vi "2 Steering Chooser.vi"() -> (2 "rudder setpoint":T2=-30.0 format="%05.1f")   [LabVIEW 2011]
doc: "Takes waypoint and boat location information from the global variable and places the approproate rudder position command on the global.\nFor Drive waypoints, this VI simply tries to make the boat's heading the same as the heading between the boat and the waypoint. TODO: this does not account for drift -- it assumes that the boat will go where it is pointed which is not always the case.\n\nTODO: important: As of 11/17 this VI only works for the Drive option.\nTODO: ideally this VI would run on any update of the boat location or waypoint location, and not otherwise."
uses:
  2 Typedefs/heading.ctl
  2 Typedefs/UTM Location.ctl
  2 Typedefs/Velocity.ctl
  2 Classes/Waypoint/Waypoint.lvclass
  2 Globals/2 Global.vi
panel:
  out "Robot UTM Location 2":T1 {"North" format="%#_10f"; "East" format="%#_8f"}
  in  "maximum rudder deflection":T2=-30.0 format="%05.1f"
  out "Robot\nHeading":T2 format="%05.1f"
  out "Angle to waypt":T2 format="%05.1f"
  out "Distance to Waypoint":T3
  out "Robot UTM Location":T1 {"North" format="%#_10f"; "East" format="%#_8f"}
  out "desired delta heading":T2 format="%05.1f"
  # "Steering Chooser simply turns the rudder to aim the boat's bow towards the next waypoint.\n\nTODO: currently only implements Drive waypoints. Also this is extremely stupid.\nImplement avoidance, stay-in-area, and maybe a PID loop."
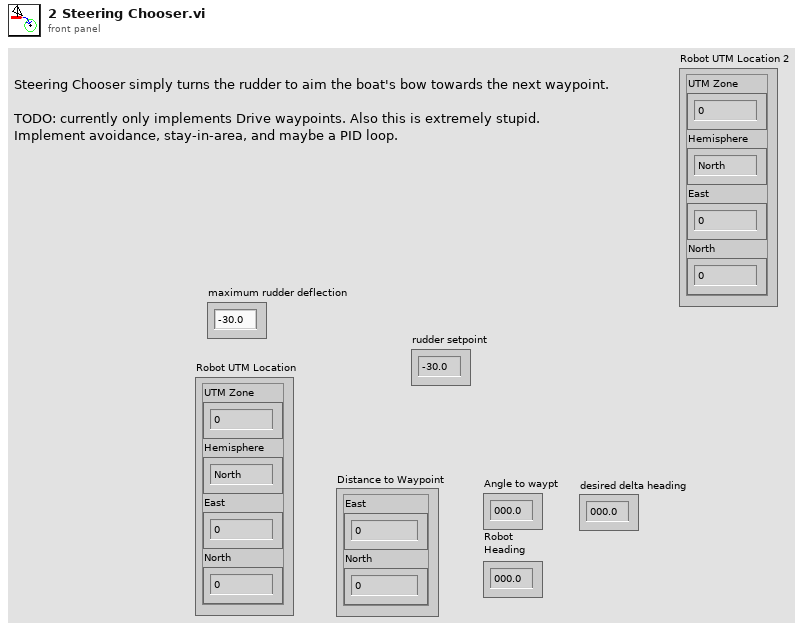
[diagram p1: front panel]
types:
  T1 = typedef "UTM Location.ctl" = cluster{"UTM Zone":dbl, "Hemisphere":enum16{"North", "South"}, "East":dbl, "North":dbl}
  T2 = typedef "heading.ctl" = dbl
  T3 = typedef "Velocity.ctl" = cluster{"East":dbl, "North":dbl}
  T4 = typedef "Current Waypoint.ctl" = i32
  T5 = typedef "Waypoints List.ctl" = refnum<class "Waypoint.lvclass">[]
  T6 = cluster{"UTM Zone":dbl, "Hemisphere":u16, "East":dbl, "North":dbl}
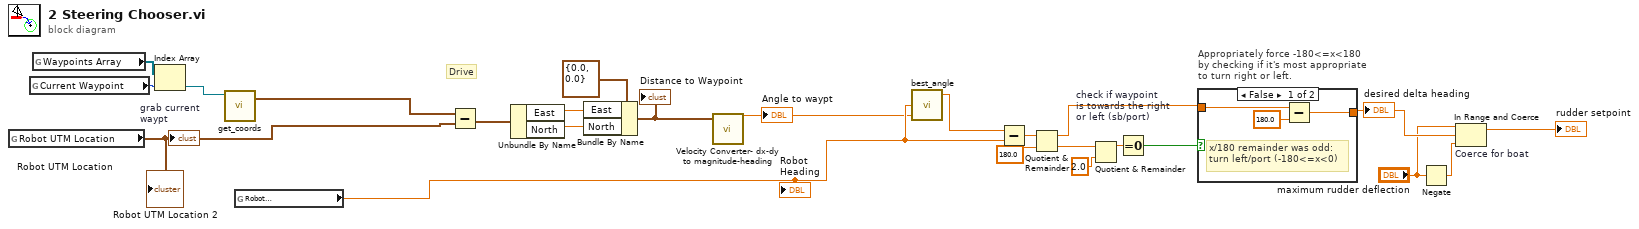
[diagram p0: block diagram]
diagram:
  # "Drive"
  n1 = global read "2 Global.vi" "Robot UTM Location"() -> (w24:T1)
  "Robot UTM Location" <- w24
  "Robot UTM Location 2" <- w24
  n2 = global read "2 Global.vi" "Current Waypoint"() -> (w21:T4)
  n3 = global read "2 Global.vi" "Waypoints Array"() -> (w22:T5)
  n4 = Index Array "grab current\nwaypt"(array=w22, index=w21) -> (element=w20:refnum<class "Waypoint.lvclass">)
  n5 = call-dynamic "get_coords.vi"("Waypoint in"=w20) -> ("Coords"=w19:T1)  [unwired: 7 in, 3 out]
  n6 = global read "2 Global.vi" "Robot\nHeading"() -> (w23:T2)
  "Robot\nHeading" <- w23
  n7 = Subtract(x=w19, y=w24) -> (x-y=w18:T6)
  n8 = Unbundle By Name(w18) -> ("East"=w17:dbl, "North"=w16:dbl)
  n9 = Bundle By Name(cluster=T3 {"East"=0.0, "North"=0.0} ("Vector In"), "East"=w17, "North"=w16) -> (w14:T3)
  "Distance to Waypoint" <- w14
  n10 = call "Velocity Converter- dx-dy to magnitude-heading.vi"("Vector In"=w14) -> ("Heading Out"=w2:T2)  [unwired: 9 in, 1 out]
  "Angle to waypt" <- w2
  n11 = call "best_angle.vi"("Waypoint Heading"=w2, "Current Heading"=w23) -> ("Best Angle"=w1:dbl)  [unwired: 1 in, 2 out]
  n12 = Subtract(x=w1, y=w23) -> (x-y=w12:T2)
  n13 = Quotient & Remainder ("shift to -180<x<180")(x=w12, y=T2 180.0) -> (x-y*floor(x/y)=w7:T2, floor(x/y)=w11:T2)
  n14 = Quotient & Remainder ("shift to -180<x<180")(x=w11, y=T2 2.0) -> (x-y*floor(x/y)=w9:T2)  [unwired: 1 out]
  n15 = Equal To 0? "check if waypoint\nis towards the right\nor left (sb/port)"(x=w9) -> (x = 0?=w8:bool)
  n16 = case "Appropriately force -180<=x<180\nby checking if it's most appropriate\nto turn right or left." shown="False" w8 {
    tunnel: w7 -> [w26 w28]
    tunnel: [w25 w28] -> w6
    frame False {
      # "x/180 remainder was odd:\nturn left/port (-180<=x<0)"
      n17 = Subtract(x=w26, y=T2 180.0) -> (x-y=w25:T2)
    }
    frame True {
      # "x/180 remainder was\neven: turn right/sb\n(0<=x<180)"
    }
  }
  "desired delta heading" <- w6
  n18 = Negate(x="maximum rudder deflection") -> (-x=w4:T2)
  n19 = In Range and Coerce "Coerce for boat"(upper limit="maximum rudder deflection", x=w6, lower limit=w4) -> (coerced(x)=→"rudder setpoint":T2)  [unwired: 1 out]
